vi "ULx Create 1D Waveform (NSamp).vi"(0 "t0":ext format="%#_10g", 5 "dt":dbl, 7 "data Array":dbl[][](array[numeric]) format="%0.2f", 9 "channelName Array":string[](array[string]), 11 "error in":errorcluster) -> (4 "data":waveform(dbl)[](array[waveform]), 15 "error out":errorcluster)   [LabVIEW 2020]
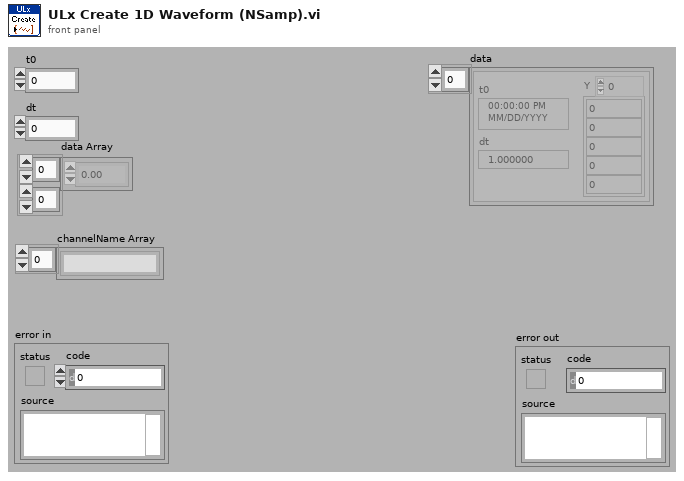
[diagram p1: front panel]
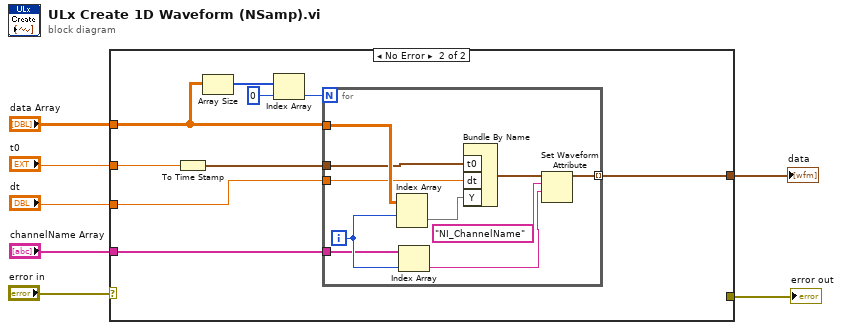
[diagram p0: block diagram]
diagram:
  n1 = case shown="No Error" "error in" {
    selector: "error in" -> [w8 _]
    tunnel: [w8 _] -> w6
    tunnel: "data Array" -> [_ w13]
    tunnel: "t0" -> [_ w12]
    tunnel: "dt" -> [_ w11]
    tunnel: "channelName Array" -> [_ w10]
    tunnel: [_ w9] -> w1
    frame Error {
    }
    frame No Error {
      n2 = To Time Stamp(1:w12) -> (0:w17:timestamp)
      n3 = Array Size(array=w13) -> (size(s)=w14:i32[])
      n4 = Index Array(array=w14, index=0) -> (element=w16:i32)
      n5 = for {
        N: w16 -> [_]
        tunnel: w13 -> [w27]
        tunnel: [w22] -> w9 mode=indexing
        tunnel: w17 -> [w25]
        tunnel: w11 -> [w24]
        tunnel: w10 -> [w18]
        i -> [w20]
        n6 = Index Array(array=w27, index (row)=w20) -> (element=w26:dbl[])  [unwired: 1 in]
        n7 = Index Array(array=w18, index=w20) -> (element=w19:string)
        n8 = Bundle By Name("t0"=w25, "dt"=w24, "Y"=w26) -> (w23:waveform(dbl))  [unwired: 1 in]
        n9 = Set Waveform Attribute(5:w19, 6:"NI_ChannelName", 7:w23) -> (3:w22:waveform(dbl))  [unwired: 1 in, 2 out]
      }
    }
  }
  "error out" <- w6
  "data" <- w1
